vi "messages_1.vi"(8 "error in (no error)":errorcluster, 9 "Data to write (no data)":bool, 10 "mesage":T1={"time stamp"=timestamp(0 s since 1904-01-01), "object"="", "header"="XX00.XX00.XX00.XX00.XX00", "message"="Z1:00000001000000000200000000030000000004000000000500000000060000000007000000000800000000092345"}, 11 "messages":refnum<queue>) -> (0 "error out":errorcluster, 3 "messages out":refnum<queue>)   [LabVIEW 2019, in "Alarms.lvlib"]
uses:
  Alarms.lvlib
  Messages/ctl/LocalMsg.ctl
  Timer Delay/format datetime 100ms.vi
  Database/PostgreSQL.lvlib
  Messages/Messages.lvlib
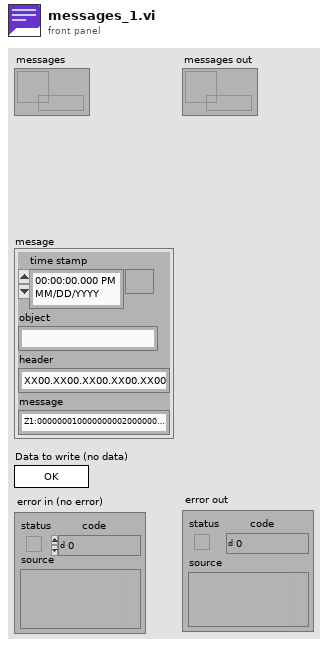
[diagram p1: front panel]
types:
  T1 = typedef "Messages.lvlib/LocalMsg.ctl" = cluster{"time stamp":timestamp, "object":string, "header":string, "message":string}
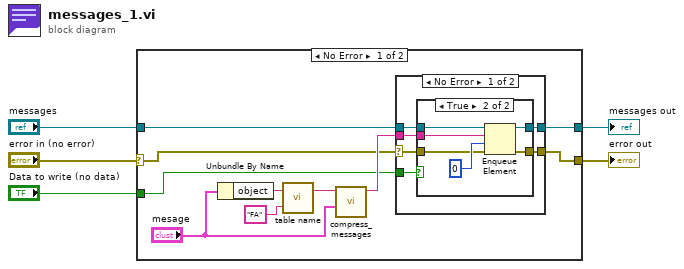
[diagram p0: block diagram]
diagram:
  n1 = case shown="No Error" "error in (no error)" {
    selector: "error in (no error)" -> [w8 w33]
    tunnel: [w12 w33] -> w4
    tunnel: [w11 w32] -> w2
    tunnel: "messages" -> [w9 w32]
    tunnel: "Data to write (no data)" -> [w10 _]
    frame No Error {
      n2 = Unbundle By Name("mesage") -> ("object"=w6:string)
      n3 = call "table name.vi"("postfix"="FA", "object name"=w6) -> ("table name"=w14:string)  [unwired: 1 in]
      n4 = call "compress_messages.vi"("mesage"="mesage", "table"=w14) -> ("message"=w13:string)  [unwired: 9 in]
      n5 = case shown="No Error" w8 {
        selector: w8 -> [w17 w31]
        tunnel: w9 -> [w21 w30]
        tunnel: w10 -> [w20 _]
        tunnel: w13 -> [w19 _]
        tunnel: [w18 w31] -> w12
        tunnel: [w16 w30] -> w11
        frame No Error {
          n6 = case shown="True" w20 {
            tunnel: w21 -> [w22 w28]
            tunnel: w19 -> [_ w27]
            tunnel: [w23 w26] -> w18
            tunnel: w17 -> [w23 w25]
            tunnel: [w22 w24] -> w16
            frame False {
            }
            frame True {
              n7 = Enqueue Element(queue=w28, element=w27, timeout in ms (-1)=0, error in (no error)=w25) -> (queue out=w24:refnum<queue>, error out=w26:errorcluster)  [unwired: 1 out]
            }
          }
        }
        frame Error {
        }
      }
    }
    frame Error {
    }
  }
  "error out" <- w4
  "messages out" <- w2
